vi "Voltage Adder.vi"() -> ()   [LabVIEW 2019]
panel:
  out "Meter":dbl(knob) scale=0.0..100.0
  in  "Numeric 3":dbl
  in  "Numeric 2":dbl
  in  "Numeric":dbl
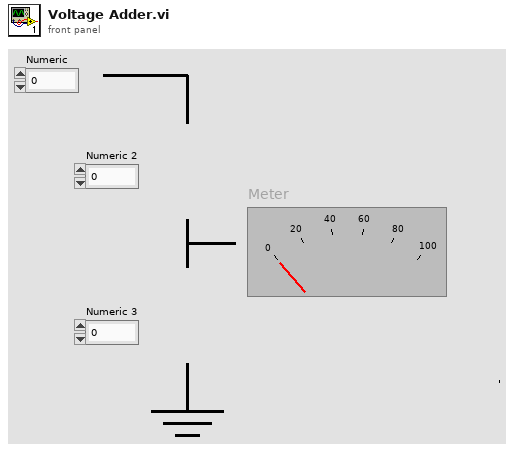
[diagram p1: front panel]
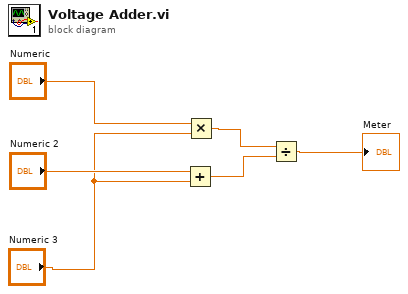
[diagram p0: block diagram]
diagram:
  n1 = Add(x="Numeric 2", y="Numeric 3") -> (x+y=w2:dbl)
  n2 = Multiply(x="Numeric", y="Numeric 3") -> (x*y=w3:dbl)
  n3 = Divide(x=w3, y=w2) -> (x/y=→"Meter":dbl)
